vi "Get Access Level.vi"(1 "Access Level Index":u16) -> (0 "Access Level Name":string)   [LabVIEW 2020]
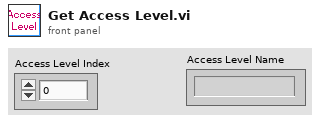
[diagram p1: front panel]
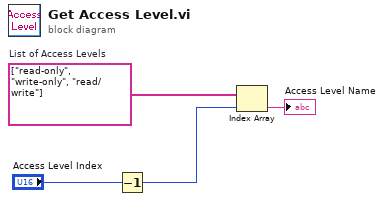
[diagram p0: block diagram]
diagram:
  w3 = string[] ["read-only", "write-only", "read/write"]  # List of Access Levels
  n1 = Decrement(x="Access Level Index") -> (x-1=w1:u16)
  n2 = Index Array(array=w3, index=w1) -> (element=→"Access Level Name":string)
